vi "Cálculos matriciais.vi"(1 "Coeficientes de controle":dbl[](array[numeric]), 2 "G":dbl, 3 "Matrizes":T3, 4 "Matriz de regularização":dbl[][](array[numeric]), 5 "Dados in":T2, 6 "E":dbl) -> (0 "Resultados":T1)   [LabVIEW 2018]
uses:
  Controles/p,q, t, a e b.ctl
  <vilib>/Analysis/baseanly.llb/A x Vector.vi
  <vilib>/Analysis/baseanly.llb/Mean (DBL).vi
  <vilib>/Analysis/baseanly.llb/Real Inverse Matrix.vi
  <vilib>/Analysis/NI_AALBase.lvlib
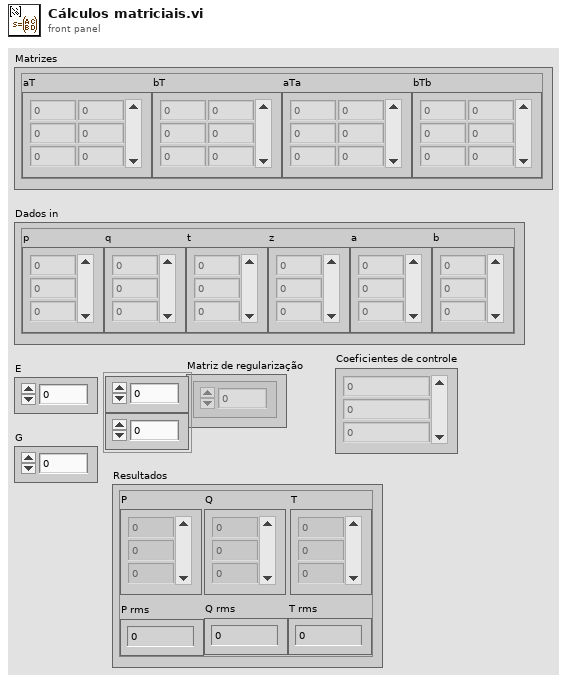
[diagram p1: front panel]
types:
  T1 = typedef "Resultados não uniformes.ctl" = cluster{"P":dbl[], "Q":dbl[], "T":dbl[], "P rms":dbl, "Q rms":dbl, "T rms":dbl}
  T2 = typedef "p,q, t, a e b.ctl" = cluster{"p":dbl[], "q":dbl[], "t":dbl[], "z":dbl[], "a":dbl[], "b":dbl[]}
  T3 = typedef "Matrizes não uniforme.ctl" = cluster{"aT":dbl[][], "bT":dbl[][], "aTa":dbl[][], "bTb":dbl[][]}
  T4 = typedef "NI_Matrix.lvlib/RealMatrix.ctl" = dbl[][]
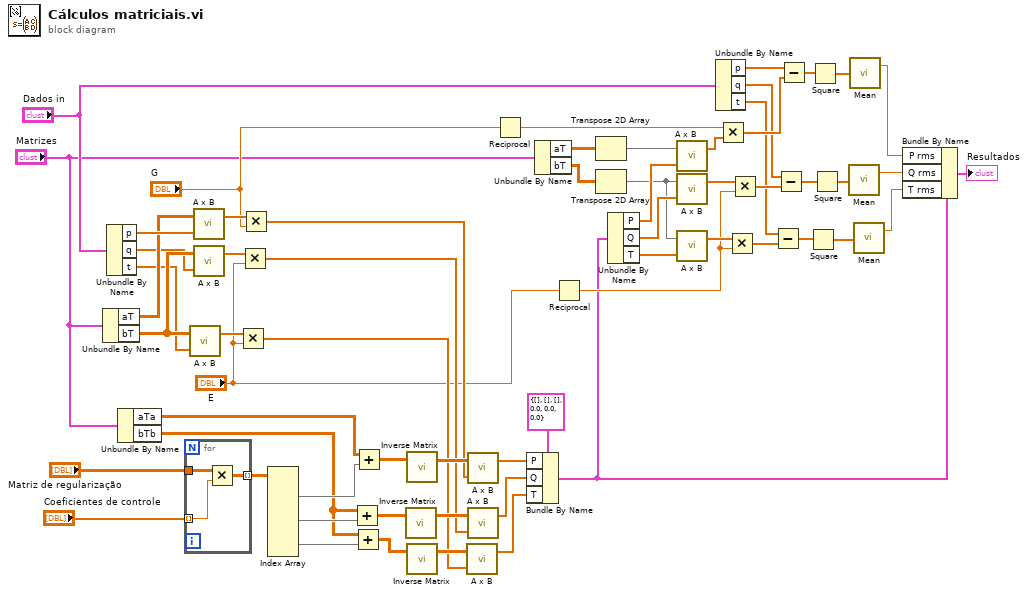
[diagram p0: block diagram]
diagram:
  n1 = Unbundle By Name("Matrizes") -> ("aT"=w44:dbl[][], "bT"=w43:dbl[][])
  n2 = Unbundle By Name("Dados in") -> ("p"=w45:dbl[], "q"=w42:dbl[], "t"=w41:dbl[])
  n3 = Unbundle By Name("Matrizes") -> ("aTa"=w57:dbl[][], "bTb"=w53:dbl[][])
  n4 = for {
    tunnel: "Coeficientes de controle" -> [w65] mode=indexing
    tunnel: "Matriz de regularização" -> [w64]
    tunnel: [w63] -> w59 mode=indexing
    n5 = Multiply(x=w64, y=w65) -> (x*y=w63:dbl[][])
  }
  n6 = call-poly <vilib>:"A x B.vi"("Vector"=w41, "A"=w43) -> ("A x Vector"=w62:dbl[])  [unwired: 1 out]
  n7 = call-poly <vilib>:"A x B.vi"("Vector"=w45, "A"=w44) -> ("A x Vector"=w49:dbl[])  [unwired: 1 out]
  n8 = call-poly <vilib>:"A x B.vi"("Vector"=w42, "A"=w43) -> ("A x Vector"=w48:dbl[])  [unwired: 1 out]
  n9 = Multiply ("Multiply.vi")(x=w62, y="E") -> (x*y=w38:dbl[])
  n10 = Multiply ("Multiply.vi")(x=w48, y="E") -> (x*y=w39:dbl[])
  n11 = Multiply ("Multiply.vi")(x=w49, y="G") -> (x*y=w40:dbl[])
  n12 = Index Array(array=w59) -> (element #1=w58:dbl[][], element #2=w54:dbl[][], element #3=w52:dbl[][])  [unwired: 9 in]
  n13 = Add(x=w53, y=w54) -> (x+y=w51:dbl[][])
  n14 = Add(x=w53, y=w52) -> (x+y=w50:dbl[][])
  n15 = Add(x=w57, y=w58) -> (x+y=w56:dbl[][])
  n16 = call-poly <vilib>:"Inverse Matrix.vi"("Input Matrix"=w51) -> ("Inverse Matrix"=w47:T4)  [unwired: 1 in, 1 out]
  n17 = call-poly <vilib>:"Inverse Matrix.vi"("Input Matrix"=w56) -> ("Inverse Matrix"=w55:T4)  [unwired: 1 in, 1 out]
  n18 = call-poly <vilib>:"Inverse Matrix.vi"("Input Matrix"=w50) -> ("Inverse Matrix"=w46:T4)  [unwired: 1 in, 1 out]
  n19 = call-poly <vilib>:"A x B.vi"("Vector"=w38, "A"=w46) -> ("A x Vector"=w34:dbl[])  [unwired: 1 out]
  n20 = call-poly <vilib>:"A x B.vi"("Vector"=w40, "A"=w55) -> ("A x Vector"=w36:dbl[])  [unwired: 1 out]
  n21 = call-poly <vilib>:"A x B.vi"("Vector"=w39, "A"=w47) -> ("A x Vector"=w35:dbl[])  [unwired: 1 out]
  n22 = Reciprocal(x="G") -> (1/x=w22:dbl)
  n23 = Bundle By Name(cluster=T1 {"P"=[], "Q"=[], "T"=[], "P rms"=0.0, "Q rms"=0.0, "T rms"=0.0} ("Resultados não uniformes"), "P"=w36, "Q"=w35, "T"=w34) -> (w6:T1)
  n24 = Unbundle By Name("Matrizes") -> ("aT"=w30:dbl[][], "bT"=w29:dbl[][])
  n25 = Reciprocal(x="E") -> (1/x=w16:dbl)
  n26 = Transpose 2D Array(2D array=w30) -> (transposed array=w28:dbl[][])
  n27 = Transpose 2D Array(2D array=w29) -> (transposed array=w24:dbl[][])
  n28 = Unbundle By Name(w6) -> ("P"=w27:dbl[], "Q"=w26:dbl[], "T"=w25:dbl[])
  n29 = call-poly <vilib>:"A x B.vi"("Vector"=w27, "A"=w28) -> ("A x Vector"=w23:dbl[])  [unwired: 1 out]
  n30 = call-poly <vilib>:"A x B.vi"("Vector"=w26, "A"=w24) -> ("A x Vector"=w18:dbl[])  [unwired: 1 out]
  n31 = call-poly <vilib>:"A x B.vi"("Vector"=w25, "A"=w24) -> ("A x Vector"=w17:dbl[])  [unwired: 1 out]
  n32 = Unbundle By Name("Dados in") -> ("p"=w21:dbl[], "q"=w13:dbl[], "t"=w1:dbl[])
  n33 = Multiply ("Multiply.vi")(x=w22, y=w23) -> (x*y=w20:dbl[])
  n34 = Multiply ("Multiply.vi")(x=w17, y=w16) -> (x*y=w14:dbl[])
  n35 = Multiply ("Multiply.vi")(x=w18, y=w16) -> (x*y=w15:dbl[])
  n36 = Subtract(x=w1, y=w14) -> (x-y=w10:dbl[])
  n37 = Subtract(x=w13, y=w15) -> (x-y=w11:dbl[])
  n38 = Subtract(x=w21, y=w20) -> (x-y=w12:dbl[])
  n39 = Square(x=w10) -> (x^2=w9:dbl[])
  n40 = Square(x=w12) -> (x^2=w7:dbl[])
  n41 = Square(x=w11) -> (x^2=w8:dbl[])
  n42 = call-poly <vilib>:"Mean.vi"("X"=w8) -> ("mean"=w4:dbl)  [unwired: 1 out]
  n43 = call-poly <vilib>:"Mean.vi"("X"=w7) -> ("mean"=w5:dbl)  [unwired: 1 out]
  n44 = call-poly <vilib>:"Mean.vi"("X"=w9) -> ("mean"=w3:dbl)  [unwired: 1 out]
  n45 = Bundle By Name(cluster=w6, "P rms"=w5, "Q rms"=w4, "T rms"=w3) -> (→"Resultados":T1)
